vi "ReadWrite CSV.vi"(6 "Task":enum16{"Save", "Read"}(ring)=enum."Read", 11 "csv?":bool) -> (3 "csv Out":bool)   [LabVIEW 2022 SP3]
panel:
  out "Pref Path":path
  out "text":string
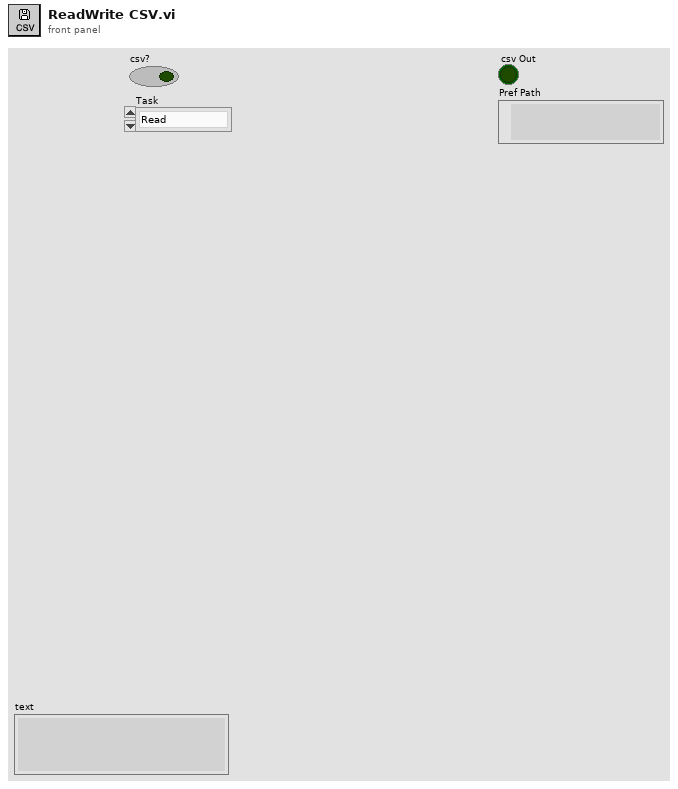
[diagram p1: front panel]
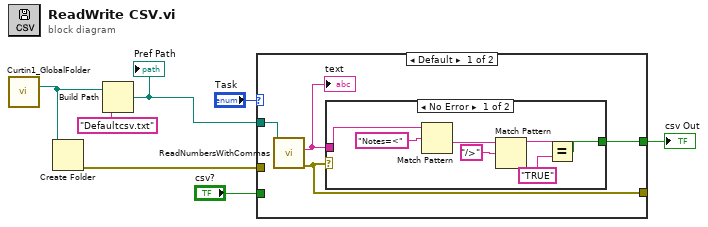
[diagram p0: block diagram]
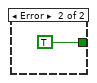
[diagram p2: hidden frame]
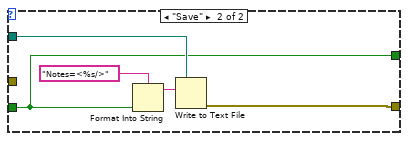
[diagram p3: hidden frame]
diagram:
  n1 = call "Curtin1_GlobalFolder.vi"() -> ("LabVIEW Data Path"=w7:path)  [unwired: 1 in, 1 out]
  n2 = Create Folder(path (use dialog)=w7) -> (error out=w6:errorcluster)  [unwired: 2 in, 2 out]
  n3 = Build Path(base path=w7, name or relative path="Defaultcsv.txt") -> (appended path=w2:path)
  "Pref Path" <- w2
  n4 = case shown="Default" "Task" {
    tunnel: "csv?" -> [_ w20]
    tunnel: w2 -> [w10 w24]
    tunnel: [w8 w21] -> _
    tunnel: [w11 w20] -> w5
    tunnel: w6 -> [_ _]
    frame Default {
      n5 = call "ReadNumbersWithCommas.vi"("file (use dialog)"=w10) -> ("error out"=w8:errorcluster, "text"=w9:string)  [unwired: 7 in, 2 out]
      "text" <- w9
      n6 = case shown="No Error" w8 {
        tunnel: [w13 TRUE] -> w11
        tunnel: w9 -> [w18 _]
        frame No Error {
          n7 = Match Pattern(string=w18, regular expression="Notes=<" ("format string")) -> (after substring=w17:string)  [unwired: 1 in, 3 out]
          n8 = Match Pattern(string=w17, regular expression="/>" ("format string")) -> (before substring=w14:string)  [unwired: 1 in, 3 out]
          n9 = Equal?(x=w14, y="TRUE" ("format string")) -> (x = y?=w13:bool)
        }
        frame Error {
        }
      }
    }
    frame "Save" {
      n10 = Format Into String(format string="Notes=<%s/>", w20) -> (resulting string=w23:string)  [unwired: 2 in, 1 out]
      n11 = Write to Text File(file (use dialog)=w24, text=w23) -> (error out=w21:errorcluster)  [unwired: 2 in, 2 out]
    }
  }
  "csv Out" <- w5
